vi "SensorColor.vi"(4 "stop":bool, 5 "Inicio":bool, 6 "Frecuencia in":bool, 7 "Frecuencia 1":bool=TRUE) -> (0 "Rojo":dbl format="%.2f", 1 "Azul":dbl, 2 "Verde":dbl format="%.2f", 3 "Sin Filtro":dbl format="%.2f")   [LabVIEW 2017]
uses:
  enumColor.ctl
  <vilib>/DAQmx/write.llb/DAQmx Write (Digital 1D Bool 1Chan 1Samp).vi
  <vilib>/DAQmx/read.llb/DAQmx Read (Counter DBL 1Chan 1Samp).vi
  <vilib>/DAQmx/create/channels.llb/DAQmx Create Channel (DO-Digital Output).vi
  <vilib>/DAQmx/create/channels.llb/DAQmx Create Channel (CI-Count Edges).vi
  <vilib>/DAQmx/miscellaneous.llb/DAQmx Fill In Error Info.vi
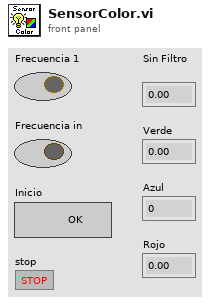
[diagram p1: front panel]
types:
  T1 = typedef "enumColor.ctl" = enum16{"Inicio", "SinFiltro1", "SinFiltro2", "SinFiltro3", "Rojo1", "Rojo2", "Rojo3", "Verde1", "Verde2", "Verde3", "Azul1", "Azul2", "Azul3", "Cierre"}
  T2 = cluster{"task out":refnum<k21>, "error out":errorcluster}
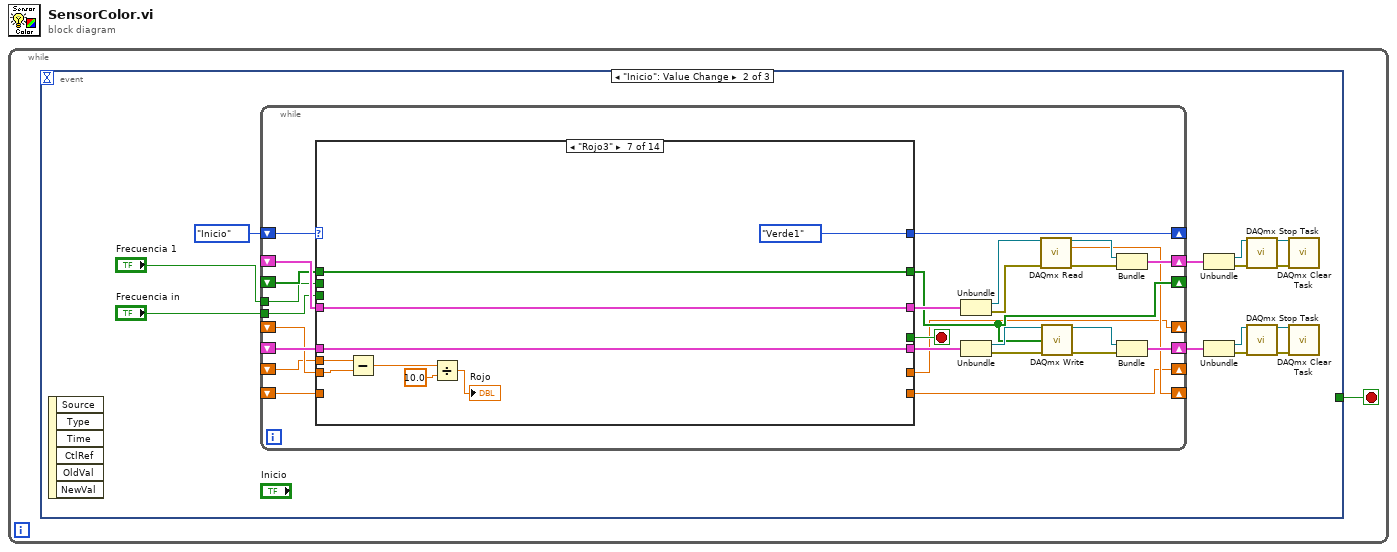
[diagram p0: block diagram]
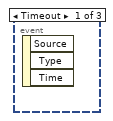
[diagram p2: hidden frame]
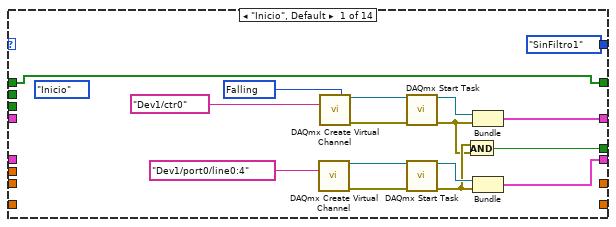
[diagram p3: hidden frame]
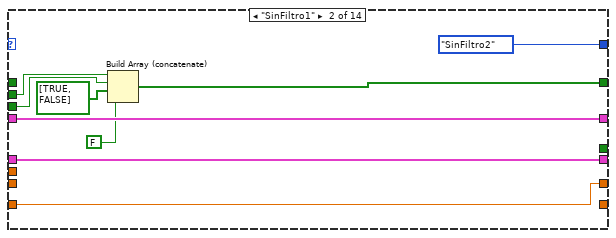
[diagram p4: hidden frame]
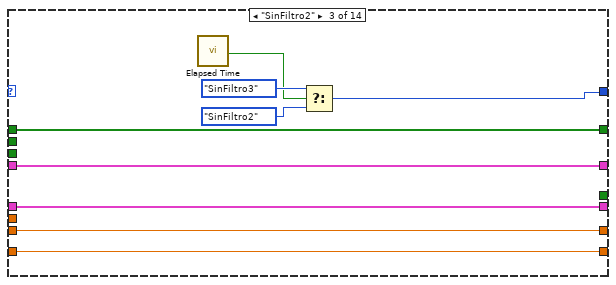
[diagram p5: hidden frame]
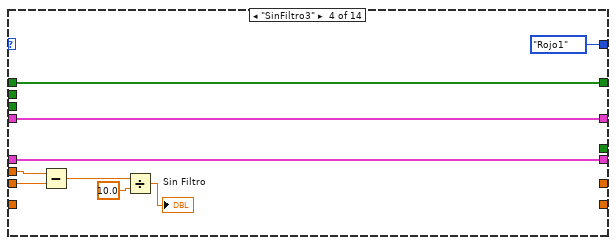
[diagram p6: hidden frame]
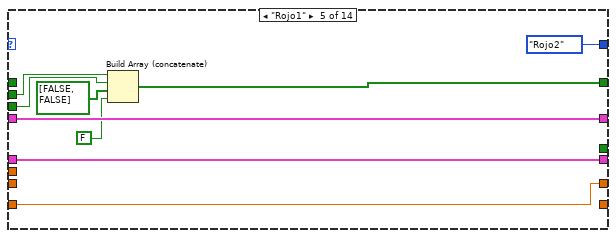
[diagram p7: hidden frame]
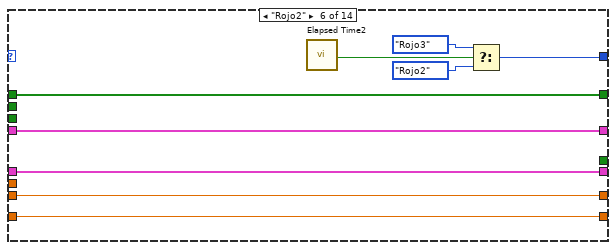
[diagram p8: hidden frame]
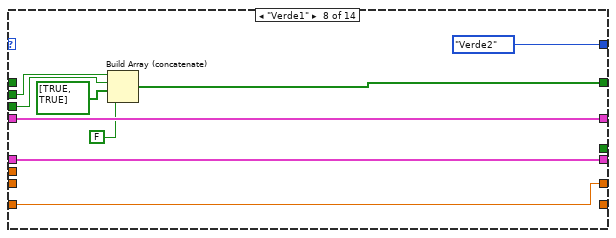
[diagram p9: hidden frame]
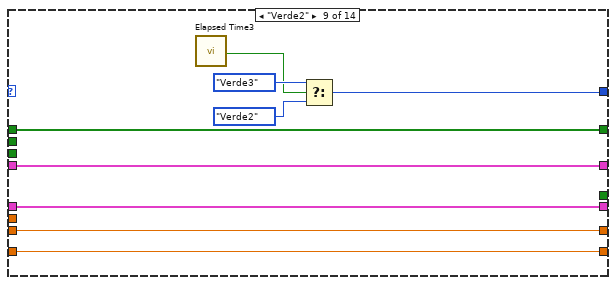
[diagram p10: hidden frame]
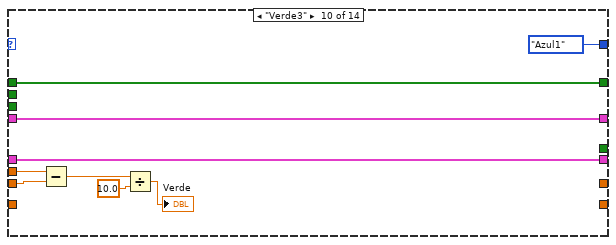
[diagram p11: hidden frame]
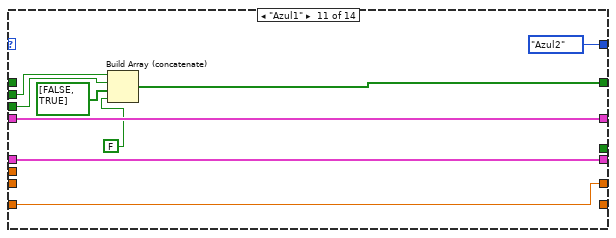
[diagram p12: hidden frame]
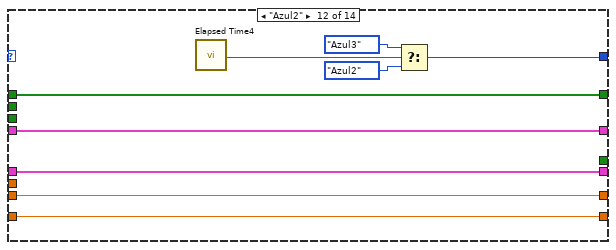
[diagram p13: hidden frame]
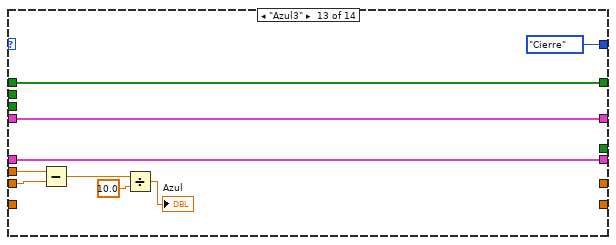
[diagram p14: hidden frame]
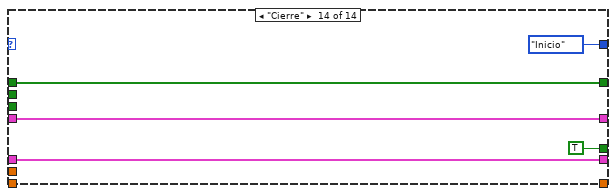
[diagram p15: hidden frame]
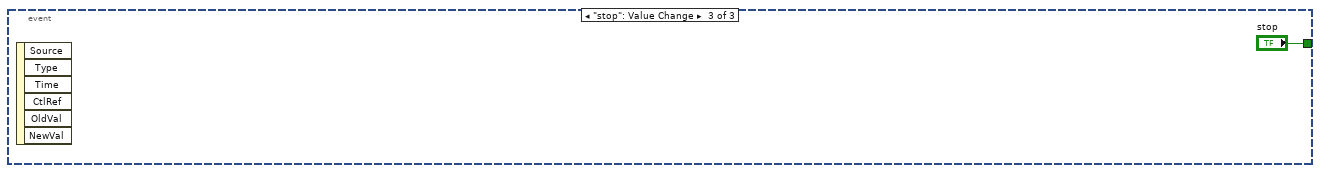
[diagram p16: hidden frame]
diagram:
  n1 = while {
    stop <- w1 stop-if-true
    n2 = event shown="[1] \"Inicio\": Value Change" {
      selector: _ -> [_ _ _]
      dyn-events: _ -> [_ _ _]
      timeout: _ -> [_ _ _]
      tunnel: [_ _ "stop"] -> w1
      event Timeout {
        n3 = event-data() -> ()  [unwired: 1 in, 3 out]
      }
      event "Inicio": Value Change {
        n4 = event-data() -> ()  [unwired: 1 in, 6 out]
        n5 = while {
          shift-right: [w40] -> _
          shift-left: enumColor."Inicio" -> [w25]
          shift-right: [w26] -> w12
          shift-left: _ -> [w27]
          shift-right: [w34] -> w11
          shift-left: _ -> [w31]
          tunnel: "Frecuencia 1" -> [w15]
          tunnel: "Frecuencia in" -> [w16]
          shift-right: [w24] -> _
          shift-left: _ -> [w23]
          shift-right: [w22] -> _
          shift-left: _ -> [w21]
          shift-right: [w20] -> _
          shift-left: _ -> [w19]
          shift-right: [w18] -> _
          shift-left: _ -> [w17]
          stop <- w41 stop-if-true
          n6 = case shown="\"Rojo3\"" w25 {
            tunnel: [w53 _ _ _ _ _ _ _ _ _ _ _ _ TRUE] -> w41
            tunnel: [w47 w66 w75 w84 w89 w102 w110 w115 w129 w137 w142 w156 w164 w169] -> w37
            tunnel: [enumColor."SinFiltro1" enumColor."SinFiltro2" w67 enumColor."Rojo1" enumColor."Rojo2" w98 enumColor."Verde1" enumColor."Verde2" w125 enumColor."Azul1" enumColor."Azul2" w152 enumColor."Cierre" enumColor."Inicio"] -> w40
            tunnel: w15 -> [_ w63 _ _ w92 _ _ w119 _ _ w146 _ _ _]
            tunnel: w16 -> [_ w62 _ _ w91 _ _ w118 _ _ w145 _ _ _]
            tunnel: [w44 w61 w74 w83 w90 w97 w109 w117 w124 w136 w144 w151 w163 w166] -> w24
            tunnel: w31 -> [_ w66 w75 w84 w89 w102 w110 w115 w129 w137 w142 w156 w164 w169]
            tunnel: [w45 w65 w73 w82 w88 w101 w111 w116 w128 w138 w143 w155 w165 w170] -> w28
            tunnel: w27 -> [_ w65 w73 w82 w88 w101 w111 w116 w128 w138 w143 w155 w165 w170]
            tunnel: w23 -> [w44 _ w74 w83 _ w97 w109 _ w124 w136 _ w151 w163 w166]
            tunnel: w21 -> [_ w59 w68 _ w86 w94 _ w113 w121 _ w141 w149 _ _]
            tunnel: [_ w59 w69 _ w86 w95 _ w113 w123 _ w141 w150 _ _] -> w20
            tunnel: w19 -> [_ _ w69 w77 _ w95 w108 _ w123 w134 _ w150 w159 _]
            tunnel: [_ _ w68 _ _ w94 _ _ w121 _ _ w149 _ _] -> w18
            tunnel: w17 -> [_ _ _ w78 _ _ w107 _ _ w135 _ _ w160 _]
            frame "Inicio", Default {
              w42 = 10171 items=["Rising"=10280, "Falling"=10171] ("edge")
              (unwired) enumColor."Inicio"
              n7 = call-poly <vilib>:"DAQmx Create Virtual Channel.vi"("lines"=tag "Dev1/port0/line0:4") -> ("task out"=w57:refnum<k21>, "error out"=w56:errorcluster)  [unwired: 13 in]
              n8 = call-poly <vilib>:"DAQmx Create Virtual Channel.vi"("edge"=w42, "counter"=tag "Dev1/ctr0") -> ("task out"=w55:refnum<k21>, "error out"=w54:errorcluster)  [unwired: 12 in]
              n9 = call <vilib>:"DAQmx Start Task.vi"("task/channels in"=w55, "error in"=w54) -> ("task out"=w49:refnum<k21>, "error out"=w48:errorcluster)  [unwired: 12 in]
              n10 = call <vilib>:"DAQmx Start Task.vi"("task/channels in"=w57, "error in"=w56) -> ("task out"=w51:refnum<k21>, "error out"=w50:errorcluster)  [unwired: 12 in]
              n11 = And(x=w50, y=w48) -> (x .and. y?=w53:bool)
              n12 = Bundle("task out"=w49, "error out"=w48) -> (w47:T2)  [unwired: 1 in]
              n13 = Bundle("task out"=w51, "error out"=w50) -> (w45:T2)  [unwired: 1 in]
            }
            frame "SinFiltro1" {
              n14 = Build Array (concatenate)(w63, w62, bool[] [TRUE, FALSE], FALSE) -> (w61:bool[])
            }
            frame "SinFiltro2" {
              n15 = call "Elapsed Time"() -> ("Time has Elapsed"=w70:bool)  [unwired: 12 in, 7 out]
              n16 = Select(t=enumColor."SinFiltro3", s=w70, f=enumColor."SinFiltro2") -> (s? t:f=w67:T1)
            }
            frame "SinFiltro3" {
              n17 = Subtract(x=w78, y=w77) -> (x-y=w81:dbl)
              n18 = Divide(x=w81, y=10.0) -> (x/y=→"Sin Filtro":dbl)
            }
            frame "Rojo1" {
              n19 = Build Array (concatenate)(w92, w91, bool[] [FALSE, FALSE], FALSE) -> (w90:bool[])
            }
            frame "Rojo2" {
              n20 = call "Elapsed Time2"() -> ("Time has Elapsed"=w96:bool)  [unwired: 12 in, 7 out]
              n21 = Select(t=enumColor."Rojo3", s=w96, f=enumColor."Rojo2") -> (s? t:f=w98:T1)
            }
            frame "Rojo3" {
              n22 = Subtract(x=w107, y=w108) -> (x-y=w106:dbl)
              n23 = Divide(x=w106, y=10.0) -> (x/y=→"Rojo":dbl)
            }
            frame "Verde1" {
              n24 = Build Array (concatenate)(w119, w118, bool[] [TRUE, TRUE], FALSE) -> (w117:bool[])
            }
            frame "Verde2" {
              n25 = call "Elapsed Time3"() -> ("Time has Elapsed"=w122:bool)  [unwired: 12 in, 7 out]
              n26 = Select(t=enumColor."Verde3", s=w122, f=enumColor."Verde2") -> (s? t:f=w125:T1)
            }
            frame "Verde3" {
              n27 = Subtract(x=w135, y=w134) -> (x-y=w132:dbl)
              n28 = Divide(x=w132, y=10.0 ("x")) -> (x/y=→"Verde":dbl)
            }
            frame "Azul1" {
              n29 = Build Array (concatenate)(w146, w145, bool[] [FALSE, TRUE], FALSE) -> (w144:bool[])
            }
            frame "Azul2" {
              n30 = call "Elapsed Time4"() -> ("Time has Elapsed"=w148:bool)  [unwired: 12 in, 7 out]
              n31 = Select(t=enumColor."Azul3", s=w148, f=enumColor."Azul2") -> (s? t:f=w152:T1)
            }
            frame "Azul3" {
              n32 = Subtract(x=w160, y=w159) -> (x-y=w161:dbl)
              n33 = Divide(x=w161, y=10.0) -> (x/y=→"Azul":dbl)
            }
            frame "Cierre" {
            }
          }
          n34 = Unbundle(w37) -> ("task out"=w36:refnum<k21>, "error out"=w35:errorcluster)
          n35 = Unbundle(w28) -> ("task out"=w39:refnum<k21>, "error out"=w38:errorcluster)
          n36 = call-poly <vilib>:"DAQmx Read.vi"("task/channels in"=w36, "error in"=w35) -> ("task out"=w33:refnum<k21>, "data"=w22:dbl, "error out"=w32:errorcluster)  [unwired: 11 in]
          n37 = call-poly <vilib>:"DAQmx Write.vi"("task/channels in"=w39, "data"=w24, "error in"=w38) -> ("task out"=w30:refnum<k21>, "error out"=w29:errorcluster)  [unwired: 10 in, 1 out]
          n38 = Bundle("task out"=w33, "error out"=w32) -> (w34:T2)  [unwired: 1 in]
          n39 = Bundle("task out"=w30, "error out"=w29) -> (w26:T2)  [unwired: 1 in]
        }
        n40 = Unbundle(w11) -> ("task out"=w8:refnum<k21>, "error out"=w7:errorcluster)
        n41 = Unbundle(w12) -> ("task out"=w10:refnum<k21>, "error out"=w9:errorcluster)
        n42 = call <vilib>:"DAQmx Stop Task.vi"("task/channels in"=w8, "error in"=w7) -> ("task out"=w4:refnum<k21>, "error out"=w3:errorcluster)  [unwired: 12 in]
        n43 = call <vilib>:"DAQmx Stop Task.vi"("task/channels in"=w10, "error in"=w9) -> ("task out"=w6:refnum<k21>, "error out"=w5:errorcluster)  [unwired: 12 in]
        n44 = call <vilib>:"DAQmx Clear Task.vi"("task in"=w4, "error in"=w3) -> ()  [unwired: 13 in, 1 out]
        n45 = call <vilib>:"DAQmx Clear Task.vi"("task in"=w6, "error in"=w5) -> ()  [unwired: 13 in, 1 out]
      }
      event "stop": Value Change {
        n46 = event-data() -> ()  [unwired: 1 in, 6 out]
      }
    }
  }
